vi "5.7-Any_UDP_Server.vi"(3 "error In":errorcluster, 4 "Data in":variant, 6 "Connection ID":refnum<k16>) -> (0 "warning out":errorcluster, 1 "data out":string, 2 "Connection ID out":refnum<k16>)   [LabVIEW 2010]
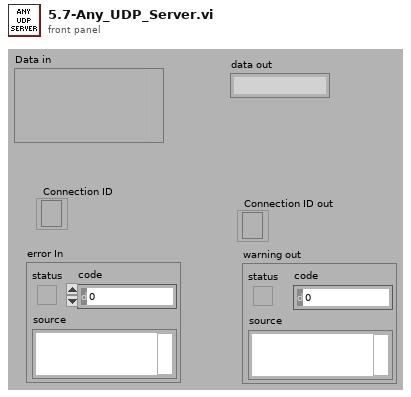
[diagram p1: front panel]
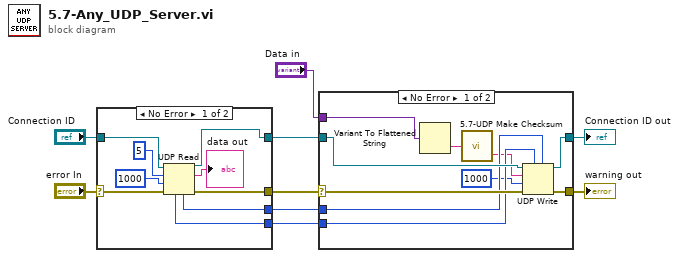
[diagram p0: block diagram]
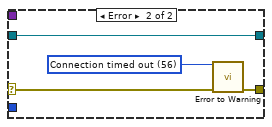
[diagram p2: hidden frame]
diagram:
  n1 = case shown="No Error" "error In" {
    selector: "error In" -> [w16 w19]
    tunnel: "Connection ID" -> [w18 w20]
    tunnel: [w15 w20] -> w4
    tunnel: [w14 w19] -> w8
    tunnel: [w12 _] -> w6
    tunnel: [w13 _] -> w5
    frame No Error {
      n2 = UDP Read(connection ID=w18, max size (548)=5, timeout ms (25000)=1000, 8:w16) -> (data out=→"data out":string, error out=w14:errorcluster, 3:w15:refnum<k16>, 4:w12:u16, 6:w13:u32)
    }
    frame Error {
    }
  }
  n3 = case shown="No Error" w8 {
    selector: w8 -> [w30 w32]
    tunnel: w4 -> [w27 w34]
    tunnel: [w29 w31] -> w7
    tunnel: [w28 w34] -> w1
    tunnel: w5 -> [w25 _]
    tunnel: w6 -> [w26 _]
    tunnel: "Data in" -> [w24 _]
    frame No Error {
      n4 = Variant To Flattened String(Variant=w24) -> (data string=w22:string)  [unwired: 1 out]
      n5 = call "5.7-UDP Make Checksum.vi"("Data String In"=w22) -> ("CS String Out"=w21:string)  [unwired: 1 out]
      n6 = UDP Write(address=w25, port or service name=w26, connection ID=w27, data in=w21, 8:w30, 9:1000 ("timeout ms (25000)")) -> (error out=w29:errorcluster, 3:w28:refnum<k16>)
    }
    frame Error {
      w33 = 56 items=["No Error", "Argument Error", "Memory Full", "Out of Zone", "End of File", "File Already Open", "Generic File IO Error", "File Not Found", "File Permission Error", "Disk Full", "Duplicate Path", "Too Many Files Open", "Not Enabled", "Resource File Not Found", "Cannot Add Resource", "Resource Not Found", "Image Not Found", "Image Memory Error", "Pen Does Not Exist", "Config Bad Type", "Config Token Not Found", "Config Parse Error", "Config Memory Error", "Bad External Code Format", "Bad External Code Offset", "External Code Not Present", "Null Window", "Destroy Window Mixup", "Null Menu", "Print Aborted", "Bad Print Record", "Print Driver Error", "Windows Error During Print", "Memory Error During Print", "Print Dialog Error", "Generic Print Error", "Invalid Device Refnum", "Device Not Found", "Device Parameter Error", "Device Unit Error", "Can't Open Device", "Device Call Aborted", "Generic Error", "Cancelled By User", "Object ID Too Low", "Object ID Too High", "Object Not In Heap", "Unknown Heap", "Bad DefProc ID", "DefProc Not In Table", "Message Out Of Range", "Null Method", "Unknown Message", "Manager Call Not Supported", "Bad address", "Connection In progress", "Connection timed out", "Connection is already in progress", "Network attribute not supported", "Network error", "Address in use", "System out of memory", "Connection aborted", "Connection refused", "Connection is not connected", "Connection is already connected", "Connection closed", "Initialize error (interapplication manager)", "Bad occurrence", "Wait on unbound occurrence handler", "Occurrence queue overflow", "Bad path", "Semaphore not signaled", "Unrecognized type (interapplication manager)"] ("1st Error to Convert")
      n7 = call <vilib>:"Error to Warning.vi"("1st Error to Convert"=w33, "error in"=w32) -> ("warning out"=w31:errorcluster)  [unwired: 13 in]
    }
  }
  "warning out" <- w7
  "Connection ID out" <- w1
